vi "testConnectTcpClient.vi"(8 "error in (no error)":errorcluster) -> (0 "error out":errorcluster, 3 "time (s)":i32)   [LabVIEW 2018]
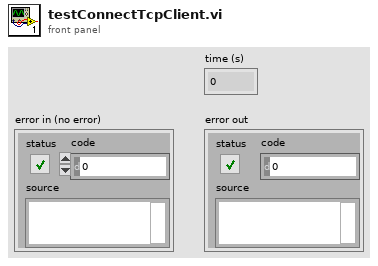
[diagram p1: front panel]
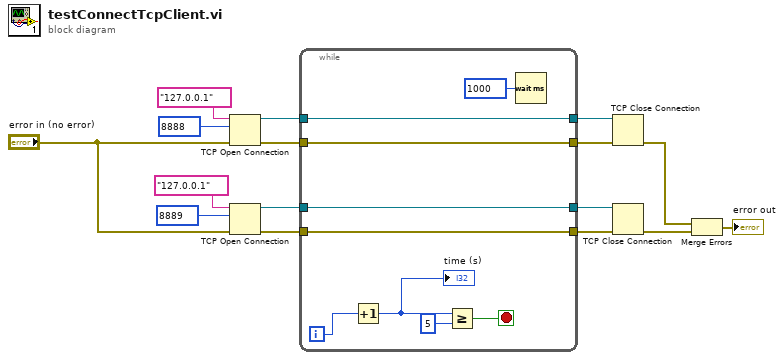
[diagram p0: block diagram]
diagram:
  n1 = TCP Open Connection(address="127.0.0.1", remote port or service name=u16 8888, error in (no error)="error in (no error)") -> (connection ID=w7:refnum<k5>, error out=w6:errorcluster)  [unwired: 2 in]
  n2 = TCP Open Connection(address="127.0.0.1", remote port or service name=u16 8889, error in (no error)="error in (no error)") -> (connection ID=w8:refnum<k5>, error out=w5:errorcluster)  [unwired: 2 in]
  n3 = while {
    tunnel: w5 -> [w19]
    tunnel: w6 -> [w20]
    tunnel: w7 -> [w21]
    tunnel: w8 -> [w18]
    tunnel: [w21] -> w9
    tunnel: [w20] -> w10
    tunnel: [w19] -> w11
    tunnel: [w18] -> w12
    i -> [w24]
    stop <- w22 stop-if-true
    n4 = Increment(x=w24) -> (x+1=w17:i32)
    "time (s)" <- w17
    n5 = Greater Or Equal?(x=w17, y=5) -> (x >= y?=w22:bool)
    n6 = Wait (ms)(milliseconds to wait=u32 1000) -> ()  [unwired: 1 out]
  }
  n7 = TCP Close Connection(connection ID=w9, error in (no error)=w10) -> (error out=w14:errorcluster)  [unwired: 1 in, 1 out]
  n8 = TCP Close Connection(connection ID=w12, error in (no error)=w11) -> (error out=w13:errorcluster)  [unwired: 1 in, 1 out]
  n9 = Merge Errors(w14, w13) -> (→"error out":errorcluster)
